vi "IMAQdxCam-Basics.vi"() -> ()   [LabVIEW 2011]
uses:
  <vilib>/vision/driver/IMAQdx.llb/IMAQdx Attribute Type.ctl
  <vilib>/vision/driver/NI_Vision_Acquisition_Software.lvlib
  C:/Program Files/National Instruments/LabVIEW 2011/resource/objmgr/imaqdx.rc
panel:
  out "Image":T1(plugin-control)
  in  "16-bit Display Mapping:Conversion Method":u32(ring)=10 items=["Default"=10, "Most Significant Bits"=11, "Full Dynamic"=12, "Downshift"=13, "Given Range"=14, "90% Dynamic"=15, "Given Percent Range"=16]
  out "LoopNo":i32
  out "error out":errorcluster
  in  "End":bool
  in  "Tab Control":enum32{"Run", "single", "startup"}(tab)=enum."startup"
  in  "Exposure":dbl(slide)=2689.598785575046 scale=100.0..100000.0
  in  "Run":bool
  in  "IMAQdx-Session":string="cam0"
  in  "AnalogGain":dbl(slide) scale=0.0..26.0
  in  "Trigger\nWait":bool
  in  "Value":dbl format="%#_9g"
  in  "Ring":u16(ring) items=["AcquisitionAttributes::AdvancedGenicam::CommandTimeout", "AcquisitionAttributes::AdvancedGenicam::EventQueueDepth", "AcquisitionAttributes::AdvancedGenicam::EventsEnabled", "AcquisitionAttributes::AdvancedGenicam::EventsSupported", "AcquisitionAttributes::Bayer::Algorithm", "AcquisitionAttributes::Bayer::GainB", "AcquisitionAttributes::Bayer::GainG", "AcquisitionAttributes::Bayer::GainR", "AcquisitionAttributes::Bayer::Pattern", "AcquisitionAttributes::ChunkDataDecoding::ChunkDataDecodingEnabled", "AcquisitionAttributes::ChunkDataDecoding::MaximumChunkCopySize", "CameraAttributes::SequencerControl::SequencerMode", "CameraAttributes::SequencerControl::SequencerSetActive", "CameraAttributes::SequencerControl::SequencerConfigurationMode", "CameraAttributes::SequencerControl::SequencerSetStart", "CameraAttributes::SequencerControl::SequencerSetSelector", "CameraAttributes::SequencerControl::SequencerSetLoad", "CameraAttributes::SequencerControl::SequencerSetSave", "CameraAttributes::SequencerControl::SequencerPathSelector", "CameraAttributes::SequencerControl::SequencerSetNext", "CameraAttributes::SequencerControl::SequencerTriggerSource", "CameraAttributes::SequencerControl::SequencerTriggerActivation", "CameraAttributes::ImageFormatControl::SensorWidth", "CameraAttributes::ImageFormatControl::SensorHeight", "CameraAttributes::ImageFormatControl::WidthMax", "CameraAttributes::ImageFormatControl::HeightMax", "CameraAttributes::ImageFormatControl::Width", "CameraAttributes::ImageFormatControl::Height", "CameraAttributes::ImageFormatControl::OffsetX", "CameraAttributes::ImageFormatControl::OffsetY", "CameraAttributes::ImageFormatControl::CenterX", "CameraAttributes::ImageFormatControl::CenterY", "CameraAttributes::ImageFormatControl::BinningHorizontalMode", "CameraAttributes::ImageFormatControl::BinningHorizontal", "CameraAttributes::ImageFormatControl::BinningVerticalMode", "CameraAttributes::ImageFormatControl::BinningVertical", "CameraAttributes::ImageFormatControl::ReverseX", "CameraAttributes::ImageFormatControl::ReverseY", "CameraAttributes::ImageFormatControl::PixelFormat", "CameraAttributes::ImageFormatControl::PixelSize", "CameraAttributes::ImageFormatControl::PixelColorFilter", "CameraAttributes::ImageFormatControl::PixelDynamicRangeMin", "CameraAttributes::ImageFormatControl::PixelDynamicRangeMax", "CameraAttributes::ImageFormatControl::TestImageSelector", "CameraAttributes::ImageFormatControl::TestImageResetAndHold", "CameraAttributes::AnalogControl::GainAuto", "CameraAttributes::AnalogControl::GainSelector", "CameraAttributes::AnalogControl::Gain", "CameraAttributes::AnalogControl::BlackLevelSelector", "CameraAttributes::AnalogControl::BlackLevel", "CameraAttributes::AnalogControl::Gamma", "CameraAttributes::AnalogControl::DigitalShift", "CameraAttributes::ImageQualityControl::PGIControl::PgiMode", "CameraAttributes::ImageQualityControl::PGIControl::NoiseReduction", "CameraAttributes::ImageQualityControl::PGIControl::SharpnessEnhancement", "CameraAttributes::ImageQualityControl::VignettingCorrectionControl::VignettingCorrectionMode", "CameraAttributes::ImageQualityControl::VignettingCorrectionControl::VignettingCorrectionLoad", "CameraAttributes::ImageQualityControl::ColorTransformationValue", "CameraAttributes::AcquisitionControl::AcquisitionMode", "CameraAttributes::AcquisitionControl::ShutterMode", "CameraAttributes::AcquisitionControl::ExposureAuto", "CameraAttributes::AcquisitionControl::ExposureMode", "CameraAttributes::AcquisitionControl::ExposureTime", "CameraAttributes::AcquisitionControl::AcquisitionBurstFrameCount", "CameraAttributes::AcquisitionControl::TriggerSelector", "CameraAttributes::AcquisitionControl::TriggerMode", "CameraAttributes::AcquisitionControl::TriggerSoftware", "CameraAttributes::AcquisitionControl::TriggerSource", "CameraAttributes::AcquisitionControl::TriggerActivation", "CameraAttributes::AcquisitionControl::TriggerDelay", "CameraAttributes::AcquisitionControl::AcquisitionFrameRateEnable", "CameraAttributes::AcquisitionControl::AcquisitionFrameRate", "CameraAttributes::AcquisitionControl::ResultingFrameRate", "CameraAttributes::AcquisitionControl::SensorReadoutTime", "CameraAttributes::AcquisitionControl::AcquisitionStatusSelector", "CameraAttributes::AcquisitionControl::AcquisitionStatus", "CameraAttributes::AutoFunctionControl::AutoTargetBrightness", "CameraAttributes::AutoFunctionControl::AutoFunctionProfile", "CameraAttributes::AutoFunctionControl::AutoGainLowerLimit", "CameraAttributes::AutoFunctionControl::AutoGainUpperLimit", "CameraAttributes::AutoFunctionControl::AutoExposureTimeLowerLimit", "CameraAttributes::AutoFunctionControl::AutoExposureTimeUpperLimit", "CameraAttributes::AutoFunctionControl::AutoFunctionROIControl::AutoFunctionROISelector", "CameraAttributes::AutoFunctionControl::AutoFunctionROIControl::AutoFunctionROIWidth", "CameraAttributes::AutoFunctionControl::AutoFunctionROIControl::AutoFunctionROIHeight", "CameraAttributes::AutoFunctionControl::AutoFunctionROIControl::AutoFunctionROIOffsetX", "CameraAttributes::AutoFunctionControl::AutoFunctionROIControl::AutoFunctionROIOffsetY", "CameraAttributes::AutoFunctionControl::AutoFunctionROIControl::AutoFunctionROIUseBrightness", "CameraAttributes::AutoFunctionControl::AutoFunctionROIControl::AutoFunctionROIUseWhiteBalance", "CameraAttributes::LUTControl::LUTSelector", "CameraAttributes::LUTControl::LUTEnable", "CameraAttributes::LUTControl::LUTIndex", "CameraAttributes::LUTControl::LUTValue", "CameraAttributes::DigitalIOControl::LineSelector", "CameraAttributes::DigitalIOControl::LineMode", "CameraAttributes::DigitalIOControl::LineFormat", "CameraAttributes::DigitalIOControl::LineLogic", "CameraAttributes::DigitalIOControl::LineSource", "CameraAttributes::DigitalIOControl::LineInverter", "CameraAttributes::DigitalIOControl::LineDebouncerTime", "CameraAttributes::DigitalIOControl::LineMinimumOutputPulseWidth", "CameraAttributes::DigitalIOControl::LineOverloadStatus", "CameraAttributes::DigitalIOControl::LineStatus", "CameraAttributes::DigitalIOControl::LineStatusAll", "CameraAttributes::DigitalIOControl::UserOutputSelector", "CameraAttributes::DigitalIOControl::UserOutputValue", "CameraAttributes::DigitalIOControl::UserOutputValueAll", "CameraAttributes::SoftwareSignalControl::SoftwareSignalSelector", "CameraAttributes::SoftwareSignalControl::SoftwareSignalPulse", "CameraAttributes::CounterAndTimerControl::TimerSelector", "CameraAttributes::CounterAndTimerControl::TimerDuration", "CameraAttributes::CounterAndTimerControl::TimerDelay", "CameraAttributes::CounterAndTimerControl::TimerTriggerSource", "CameraAttributes::CounterAndTimerControl::CounterSelector", "CameraAttributes::CounterAndTimerControl::CounterEventSource", "CameraAttributes::CounterAndTimerControl::CounterResetSource", "CameraAttributes::CounterAndTimerControl::CounterResetActivation", "CameraAttributes::CounterAndTimerControl::CounterReset", "CameraAttributes::CounterAndTimerControl::CounterDuration", "CameraAttributes::BslLightControl::BslLightControlMode", "CameraAttributes::BslLightControl::BslLightControlSource", "CameraAttributes::BslLightControl::BslLightControlEnumerateDevices", "CameraAttributes::BslLightControl::BslLightControlStatus", "CameraAttributes::BslLightControl::BslLightControlErrorStatus", "CameraAttributes::BslLightControl::BslLightControlTriggerMode", "CameraAttributes::BslLightControl::BslLightDeviceSelector", "CameraAttributes::BslLightControl::BslLightDeviceMaxCurrent", "CameraAttributes::BslLightControl::BslLightDeviceBrightness", "CameraAttributes::BslLightControl::BslLightDeviceOperationMode", "CameraAttributes::BslLightControl::BslLightDeviceStrobeMode", "CameraAttributes::BslLightControl::BslLightDeviceStrobeDuration", "CameraAttributes::BslLightControl::BslLightDeviceLastError", "CameraAttributes::BslLightControl::BslLightDeviceClearLastError", "CameraAttributes::BslLightControl::BslLightDeviceChangeID", "CameraAttributes::BslLightControl::BslLightDeviceFirmwareVersion", "CameraAttributes::ChunkDataControl::ChunkModeActive", "CameraAttributes::ChunkDataControl::ChunkSelector", "CameraAttributes::ChunkDataControl::ChunkEnable", "CameraAttributes::ChunkDataControl::ChunkGainSelector", "CameraAttributes::ChunkDataControl::ChunkGain", "CameraAttributes::ChunkDataControl::ChunkExposureTime", "CameraAttributes::ChunkDataControl::ChunkTimestamp", "CameraAttributes::ChunkDataControl::ChunkLineStatusAll", "CameraAttributes::ChunkDataControl::ChunkCounterSelector", "CameraAttributes::ChunkDataControl::ChunkCounterValue", "CameraAttributes::ChunkDataControl::ChunkSequencerSetActive", "CameraAttributes::ChunkDataControl::ChunkPayloadCRC16", "CameraAttributes::ChunkDataControl::ChunkData::ChunkGainSelector", "CameraAttributes::ChunkDataControl::ChunkData::ChunkGain", "CameraAttributes::ChunkDataControl::ChunkData::ChunkExposureTime", "CameraAttributes::ChunkDataControl::ChunkData::ChunkTimestamp", "CameraAttributes::ChunkDataControl::ChunkData::ChunkLineStatusAll", "CameraAttributes::ChunkDataControl::ChunkData::ChunkCounterSelector", "CameraAttributes::ChunkDataControl::ChunkData::ChunkCounterValue", "CameraAttributes::ChunkDataControl::ChunkData::ChunkSequencerSetActive", "CameraAttributes::ChunkDataControl::ChunkData::ChunkPayloadCRC16", "CameraAttributes::EventControl::EventSelector", "CameraAttributes::EventControl::EventNotification", "CameraAttributes::EventControl::EventExposureEndData::EventExposureEnd", "CameraAttributes::EventControl::EventExposureEndData::EventExposureEndTimestamp", "CameraAttributes::EventControl::EventExposureEndData::EventExposureEndFrameID", "CameraAttributes::EventControl::EventFrameBurstStartData::EventFrameBurstStart", "CameraAttributes::EventControl::EventFrameBurstStartData::EventFrameBurstStartTimestamp", "CameraAttributes::EventControl::EventFrameBurstStartData::EventFrameBurstStartFrameID", "CameraAttributes::EventControl::EventFrameStartOvertriggerData::EventFrameStartOvertrigger", "CameraAttributes::EventControl::EventFrameStartOvertriggerData::EventFrameStartOvertriggerTimestamp", "CameraAttributes::EventControl::EventFrameStartOvertriggerData::EventFrameStartOvertriggerFrameID", "CameraAttributes::EventControl::EventFrameBurstStartOvertriggerData::EventFrameBurstStartOvertrigger", "CameraAttributes::EventControl::EventFrameBurstStartOvertriggerData::EventFrameBurstStartOvertriggerTimestamp", "CameraAttributes::EventControl::EventFrameBurstStartOvertriggerData::EventFrameBurstStartOvertriggerFrameID", "CameraAttributes::EventControl::EventCriticalTemperatureData::EventCriticalTemperature", "CameraAttributes::EventControl::EventCriticalTemperatureData::EventCriticalTemperatureTimestamp", "CameraAttributes::EventControl::EventOverTemperatureData::EventOverTemperature", "CameraAttributes::EventControl::EventOverTemperatureData::EventOverTemperatureTimestamp", "CameraAttributes::EventControl::EventFrameStartWaitData::EventFrameStartWait", "CameraAttributes::EventControl::EventFrameStartWaitData::EventFrameStartWaitTimestamp", "CameraAttributes::EventControl::EventFrameBurstStartWaitData::EventFrameBurstStartWait", "CameraAttributes::EventControl::EventFrameBurstStartWaitData::EventFrameBurstStartWaitTimestamp", "CameraAttributes::UserSetControl::UserSetSelector", "CameraAttributes::UserSetControl::UserSetLoad", "CameraAttributes::UserSetControl::UserSetSave", "CameraAttributes::UserSetControl::UserSetDefault", "CameraAttributes::TransportLayerControl::PayloadSize", "CameraAttributes::TransportLayerControl::BslUSBSpeedMode", "CameraAttributes::TransportLayerControl::SIPayloadTransferSize", "CameraAttributes::TransportLayerControl::SIPayloadTransferCount", "CameraAttributes::TransportLayerControl::SIPayloadFinalTransfer1Size", "CameraAttributes::TransportLayerControl::SIPayloadFinalTransfer2Size", "CameraAttributes::DeviceControl::DeviceVendorName", "CameraAttributes::DeviceControl::DeviceModelName", "CameraAttributes::DeviceControl::DeviceManufacturerInfo", "CameraAttributes::DeviceControl::DeviceVersion", "CameraAttributes::DeviceControl::DeviceFirmwareVersion", "CameraAttributes::DeviceControl::DeviceSerialNumber", "CameraAttributes::DeviceControl::DeviceUserID", "CameraAttributes::DeviceControl::DeviceScanType", "CameraAttributes::DeviceControl::TimestampLatch", "CameraAttributes::DeviceControl::TimestampLatchValue", "CameraAttributes::DeviceControl::DeviceLinkSelector", "CameraAttributes::DeviceControl::DeviceLinkSpeed", "CameraAttributes::DeviceControl::DeviceLinkThroughputLimitMode", "CameraAttributes::DeviceControl::DeviceLinkThroughputLimit", "CameraAttributes::DeviceControl::DeviceLinkCurrentThroughput", "CameraAttributes::DeviceControl::DeviceTemperatureSelector", "CameraAttributes::DeviceControl::DeviceTemperature", "CameraAttributes::DeviceControl::TemperatureState", "CameraAttributes::DeviceControl::DeviceSFNCVersionMajor", "CameraAttributes::DeviceControl::DeviceSFNCVersionMinor", "CameraAttributes::DeviceControl::DeviceSFNCVersionSubMinor", "CameraAttributes::UserDefinedValueControl::UserDefinedValueSelector", "CameraAttributes::UserDefinedValueControl::UserDefinedValue", "CameraAttributes::RemoveParameterLimitControl::RemoveParameterLimitSelector", "CameraAttributes::RemoveParameterLimitControl::RemoveParameterLimit", "CameraAttributes::ExpertFeatureAccess::ExpertFeatureAccessSelector", "CameraAttributes::ExpertFeatureAccess::ExpertFeatureAccessKey", "CameraAttributes::ExpertFeatureAccess::ExpertFeatureEnable", "CameraAttributes::FileAccessControl::FileSelector", "CameraAttributes::FileAccessControl::FileOperationSelector", "CameraAttributes::FileAccessControl::FileOpenMode", "CameraAttributes::FileAccessControl::FileAccessOffset", "CameraAttributes::FileAccessControl::FileAccessLength", "CameraAttributes::FileAccessControl::FileOperationStatus", "CameraAttributes::FileAccessControl::FileOperationResult", "CameraAttributes::FileAccessControl::FileSize", "CameraAttributes::FileAccessControl::FileOperationExecute", "AcquisitionAttributes::BitsPerPixel", "AcquisitionAttributes::ImageDecoderCopyMode", "AcquisitionAttributes::IncompleteBufferMode", "AcquisitionAttributes::OutputImageType", "AcquisitionAttributes::OverwriteMode", "AcquisitionAttributes::ReceiveTimestampMode", "AcquisitionAttributes::ShiftPixelBits", "AcquisitionAttributes::SwapPixelBytes", "AcquisitionAttributes::Timeout", "CameraInformation::BaseAddress", "CameraInformation::BusType", "CameraInformation::ModelName", "CameraInformation::PrimaryURLString", "CameraInformation::SecondaryURLString", "CameraInformation::SerialNumberHigh", "CameraInformation::SerialNumberLow", "CameraInformation::USBConnectionSpeed", "CameraInformation::VendorName", "StatusInformation::AcqInProgress", "StatusInformation::HandledEventCount", "StatusInformation::IncompleteBufferCount", "StatusInformation::LastBufferCount", "StatusInformation::LastBufferNumber", "StatusInformation::LostBufferCount", "StatusInformation::LostEventCount"]
  out "Description":string
  out "IsWritable":bool
  out "Attribute Type":T2=enum."Bool"
  in  "IMAQdx-start":string
  out "initerror":errorcluster
  # "init an test the cam with NiMax first! Find Session name"
  # "! Space nach name und type vor komma\nName, \nType[U32,I64,DBL,String,Enum,Bool,Command], \nRead, \nWrite[0,1], \nValue"
  # "init the cam in MAX first!"
  # "read"
  # "change=write"
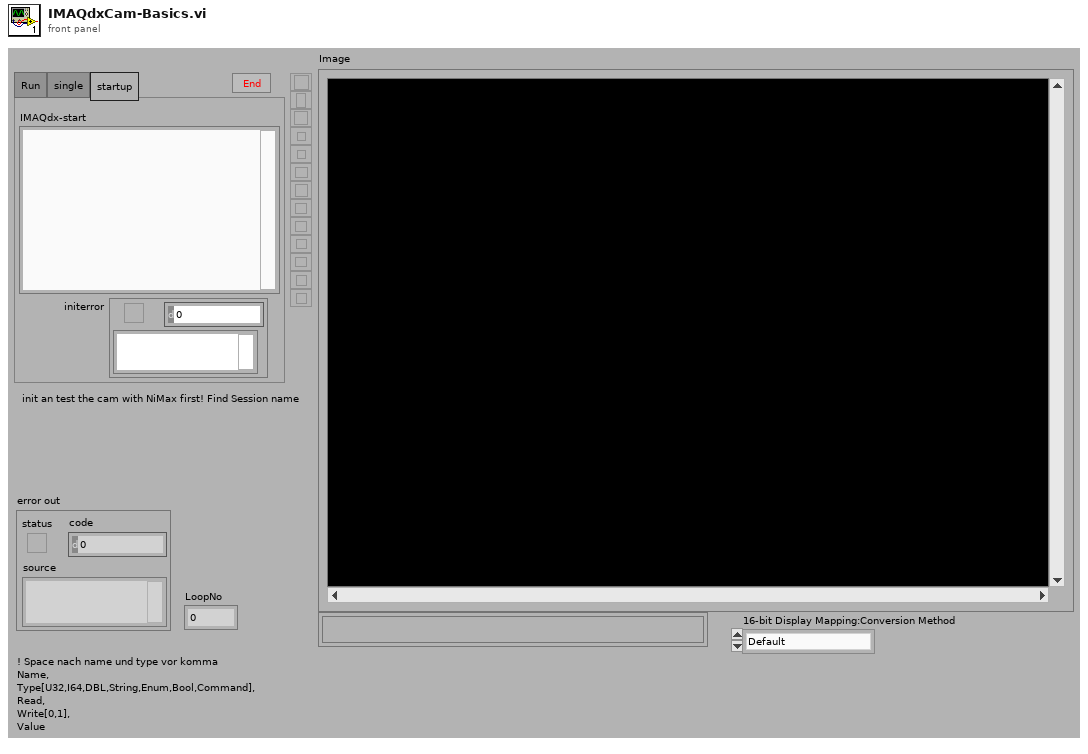
[diagram p1: front panel]
types:
  T1 = typedef "IMAQ Image.ctl" = refnum<image>
  T2 = typedef "NI_Vision_Acquisition_Software.lvlib/IMAQdx Attribute Type.ctl" = enum32{"U32", "I64", "DBL", "String", "Enum", "Bool", "Command"}
  T3 = typedef "Image Type" = u32
  T4 = typedef "IMAQdx.ctl" = refnum<k21>
  T5 = cluster{"Attribute Type":T2, "Readable":bool, "Writable":bool, "Attribute Name":string}[]
  T6 = cluster{"Global Rectangle":i32[], "Contours":cluster{"Contour Type":u32, "ROI Type":u32, "Points":i32[]}[]}
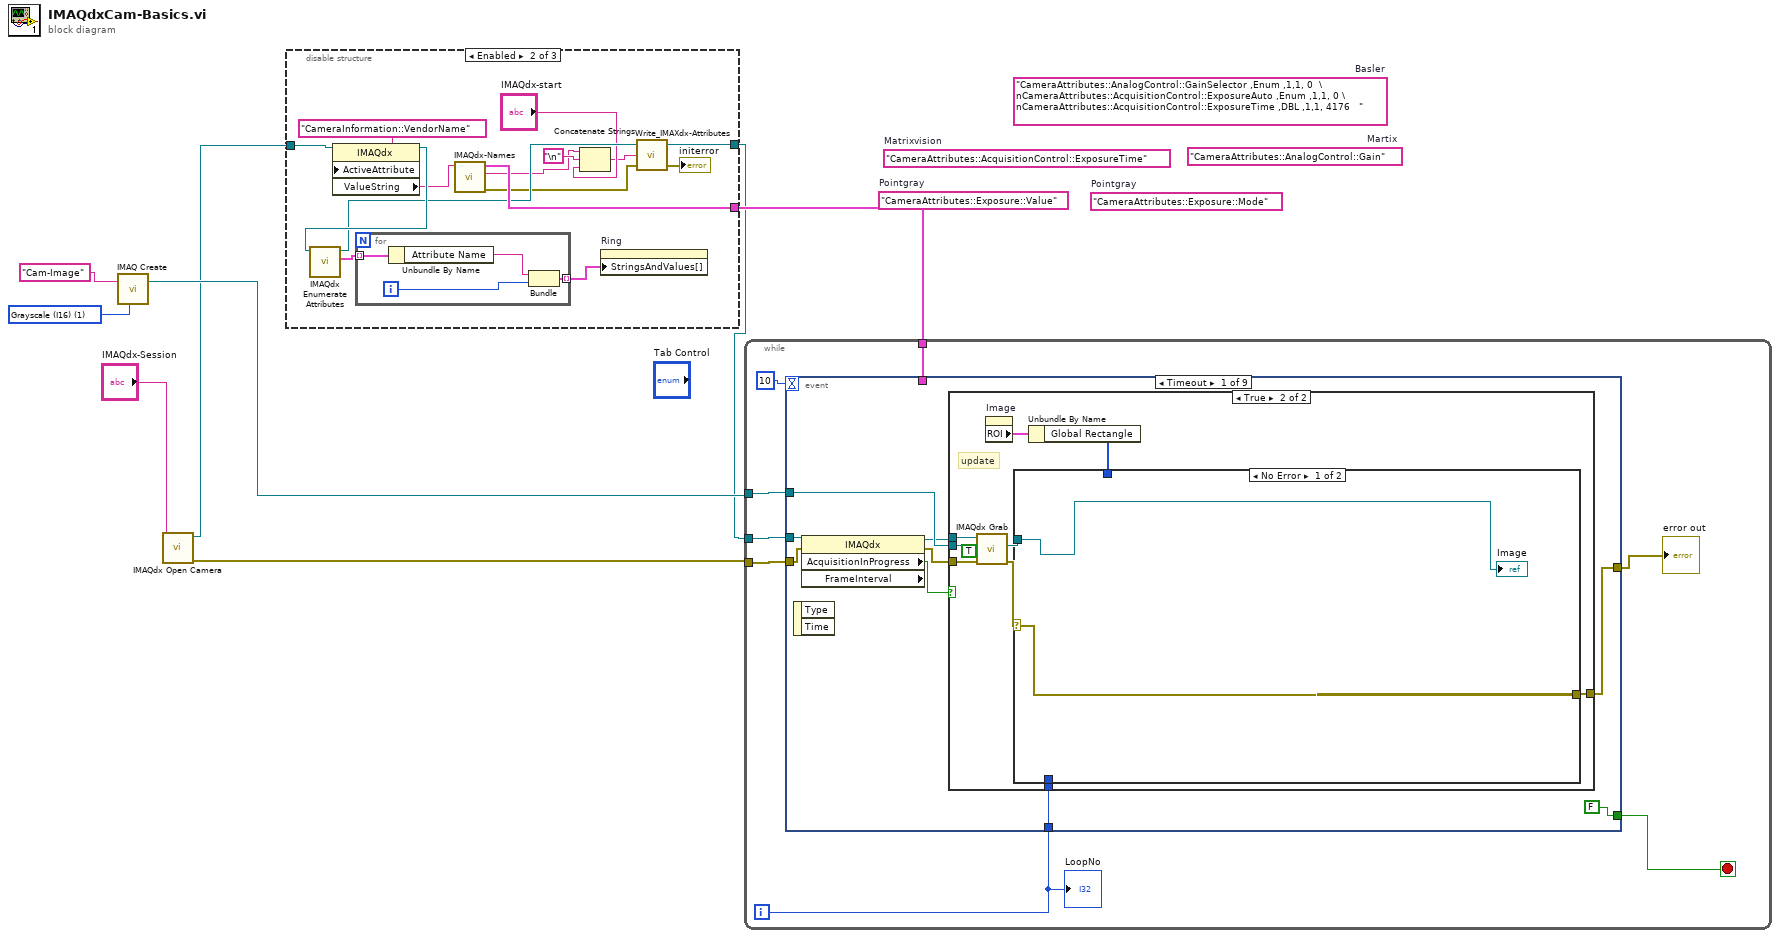
[diagram p0: block diagram]
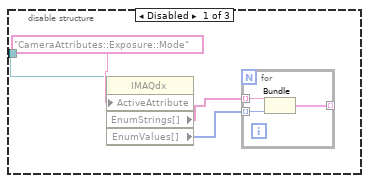
[diagram p2: hidden frame]
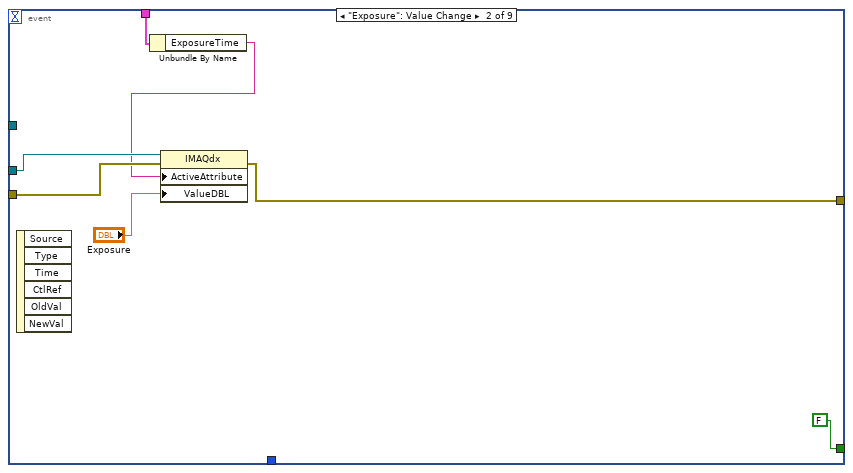
[diagram p6: hidden frame]
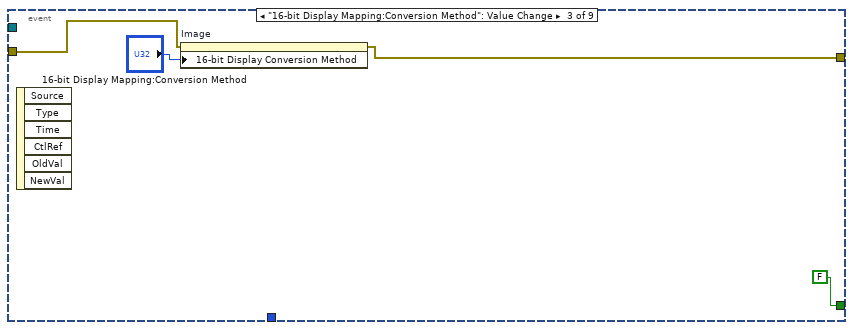
[diagram p7: hidden frame]
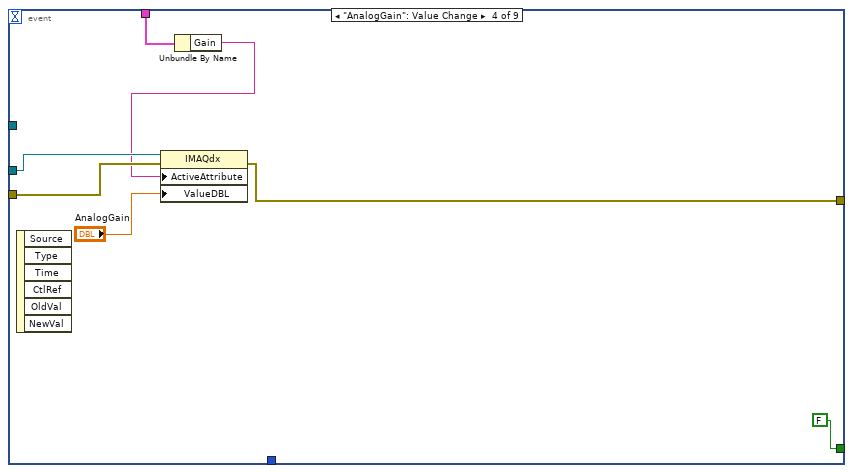
[diagram p8: hidden frame]
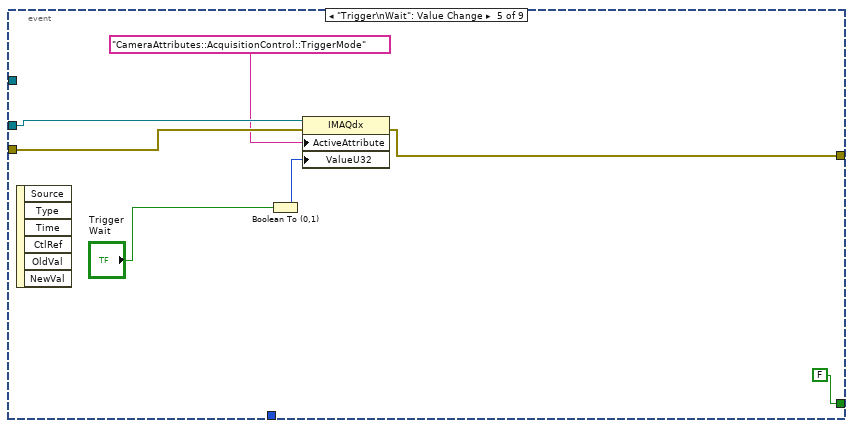
[diagram p9: hidden frame]
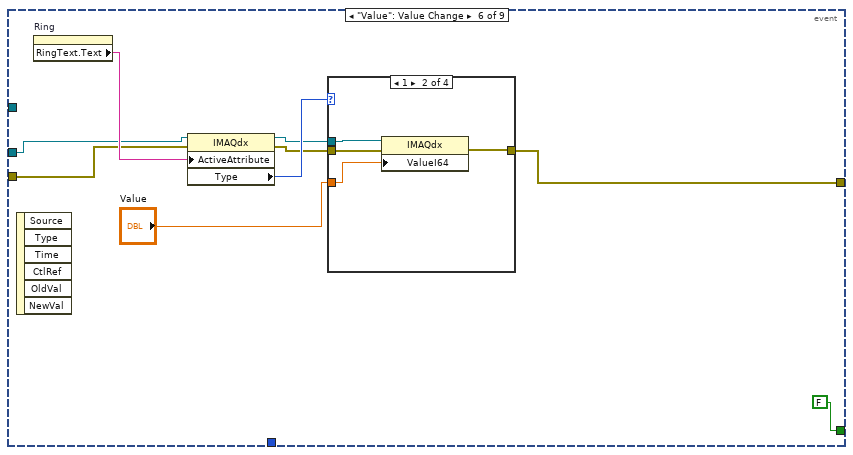
[diagram p10: hidden frame]
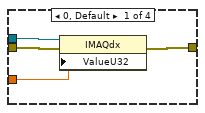
[diagram p11: hidden frame]
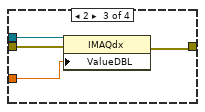
[diagram p12: hidden frame]
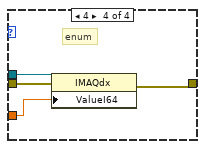
[diagram p13: hidden frame]
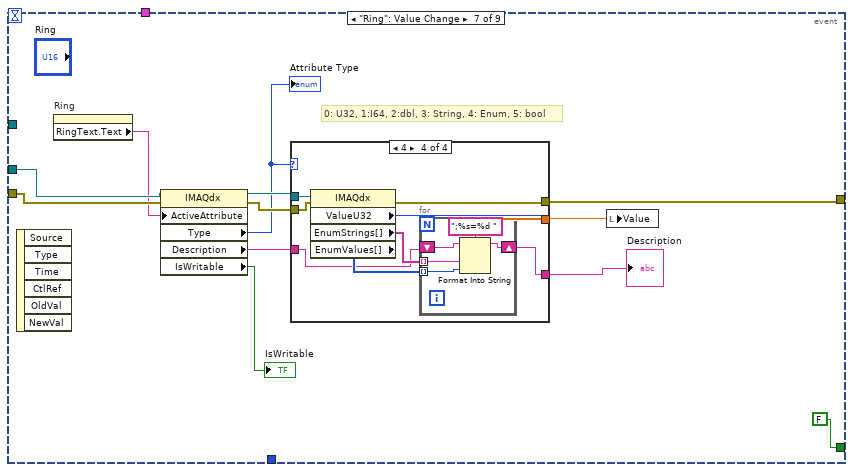
[diagram p14: hidden frame]
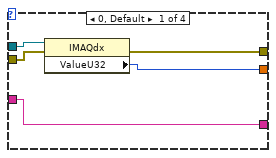
[diagram p15: hidden frame]
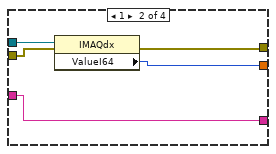
[diagram p16: hidden frame]
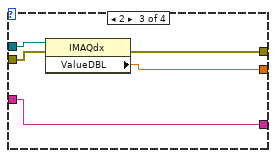
[diagram p17: hidden frame]
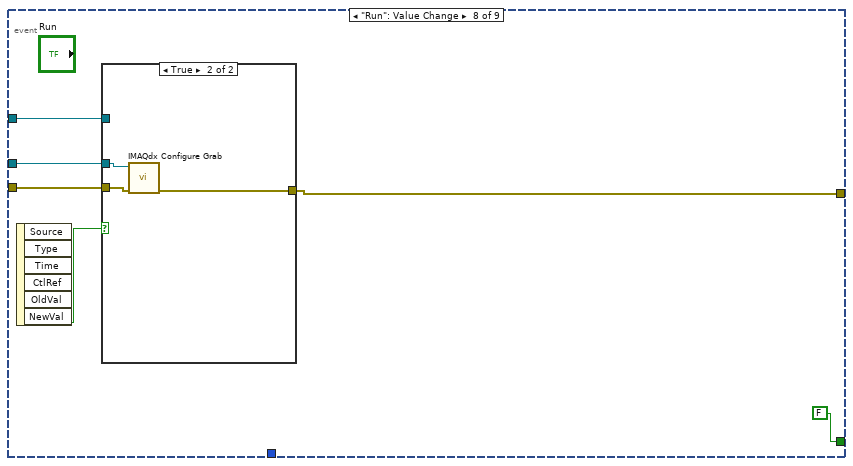
[diagram p18: hidden frame]
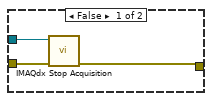
[diagram p19: hidden frame]
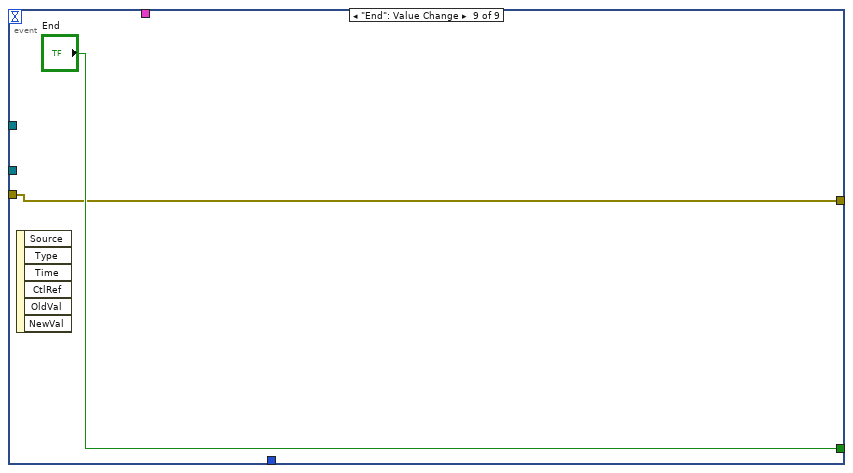
[diagram p20: hidden frame]
diagram:
  (unwired) "CameraAttributes::AnalogControl::Gain"  # Martix
  (unwired) "CameraAttributes::AnalogControl::GainSelector ,Enum ,1,1, 0  \nCameraAttributes::AcquisitionControl::ExposureAuto ,Enum ,1,1, 0 \nCameraAttributes::AcquisitionControl::ExposureTime ,DBL ,1,1, 4176   "  # Basler
  (unwired) "CameraAttributes::Exposure::Mode"  # Pointgray
  (unwired) "CameraAttributes::Exposure::Value"  # Pointgray
  (unwired) "CameraAttributes::AcquisitionControl::ExposureTime"  # Matrixvision
  w3 = T3 1 items=["Grayscale (U8)", "Grayscale (I16)", "Grayscale (SGL)", "Complex (CSG)", "RGB (U32)", "HSL (U32)", "RGB (U64)", "Grayscale (U16)"] ("Image Type")
  n1 = call "IMAQ Create"("Image Name"="Cam-Image", "Image Type"=w3) -> ("New Image"=w6:T1)  [unwired: 2 in, 2 out]
  n2 = call <vilib>:"IMAQdx Open Camera.vi"("Session In"="IMAQdx-Session") -> ("error out"=w7:errorcluster, "Session Out"=w5:T4)  [unwired: 2 in, 7 out]
  n3 = disable-structure shown="Enabled" {
    disable-tunnel: w5 -> [w11 w28 w35]
    disable-tunnel: [_ w24 _] -> w2
    disable-tunnel: [_ w22 w35] -> w1
    frame Disabled {
      n4 = property class="IMAQdx"(reference=w11, "ActiveAttribute"="CameraAttributes::Exposure::Mode" ("Attribute Name")) -> ("EnumStrings[]"=w10:string[], "EnumValues[]"=w9:u32[])  [unwired: 1 in, 2 out]
      n5 = for {
        tunnel: w10 -> [w15] mode=indexing
        tunnel: w9 -> [w14] mode=indexing
        tunnel: [w13] -> _ mode=indexing
        n6 = Bundle(w15, w14) -> (w13:cluster{string, u32})  [unwired: 1 out]
      }
    }
    frame Enabled {
      n7 = property class="IMAQdx"(reference=w28, "ActiveAttribute"="CameraInformation::VendorName") -> (reference out=w26:T4, "ValueString"=w25:string)  [unwired: 1 in, 1 out]
      n8 = call <vilib>:"IMAQdx Enumerate Attributes.vi"("Session In"=w26) -> ("Attribute Information Array"=w27:T5, "Session Out"=w23:T4)  [unwired: 8 in, 1 out]
      n9 = for {
        tunnel: w27 -> [w34] mode=indexing
        tunnel: [w31] -> w29 mode=indexing
        i -> [w32]
        n10 = Unbundle By Name(w34) -> ("Attribute Name"=w33:string)
        n11 = Bundle("Attribute Name"=w33, w32) -> (w31:cluster{"Attribute Name":string, i32})  [unwired: 1 in]
      }
      n12 = call "IMAQdx-Names.vi"("exactCameraName"=w25) -> ("error out"=w16:errorcluster, "Defaults"=w20:string, "shortcuts"=w24:cluster{"ExposureTime":string, "Gain":string})  [unwired: 8 in]
      n13 = Concatenate Strings(w20, "\n", "IMAQdx-start") -> (w18:string)
      n14 = property on="Ring" class="Ring (strict)"("StringsAndValues[]"=w29) -> ()  [unwired: 2 in, 2 out]
      n15 = call "Write_IMAXdx-Attributes.vi"("error in"=w16, "IMAQdx-Defaults"=w18, "Session In"=w23) -> ("error out"=→"initerror":errorcluster, "Session Out"=w22:T4)  [unwired: 1 in]
    }
    frame Disabled {
    }
  }
  n16 = while {
    tunnel: w1 -> [w43]
    tunnel: w7 -> [w42]
    tunnel: w6 -> [w41]
    tunnel: w2 -> [w36]
    i -> [w37]
    stop <- w40 stop-if-true
    n17 = event shown="[0] Timeout" {
      selector: _ -> [_ _ _ _ _ _ _ _ _]
      dyn-events: _ -> [_ _ _ _ _ _ _ _ _]
      timeout: 10 -> [_ _ _ _ _ _ _ _ _]
      tunnel: w43 -> [w48 w72 _ w84 w89 w96 w126 w161 _]
      tunnel: w42 -> [w47 w71 w75 w83 w88 w94 w124 w160 w169]
      tunnel: w41 -> [w52 _ _ _ _ _ _ w159 _]
      tunnel: [FALSE ("End") FALSE ("End") FALSE ("End") FALSE ("End") FALSE ("End") FALSE ("End") FALSE ("End") FALSE ("End") "End"] -> w40
      tunnel: [w49 w70 w74 w82 w86 w100 w128 w158 w169] -> w38
      tunnel: w37 -> [w45 _ _ _ _ _ _ _ _]
      tunnel: w36 -> [_ w69 _ w81 _ _ _ _ _]
      event Timeout {
        n18 = event-data() -> ()  [unwired: 3 out]
        n19 = property class="IMAQdx" props=["AcquisitionInProgress", "FrameInterval"](reference=w48, error in=w47) -> (reference out=w50:T4, error out=w46:errorcluster, "AcquisitionInProgress"=w51:bool)  [unwired: 1 out]
        n20 = case shown="True" w51 {
          tunnel: w52 -> [_ w63]
          tunnel: w46 -> [w53 w62]
          tunnel: w50 -> [_ w61]
          tunnel: [w53 w57] -> w49
          tunnel: w45 -> [_ w58]
          frame False {
          }
          frame True {
            # "update"
            n21 = call <vilib>:"IMAQdx Grab.vi"("error in"=w62, "Wait for Next Buffer? (Yes)"=TRUE, "Image In"=w63, "Session In"=w61) -> ("error out"=w55:errorcluster, "Image Out"=w59:T1)  [unwired: 6 out]
            n22 = property on="Image" class="ImageControl"() -> ("ROI"=w54:T6)  [unwired: 2 in, 2 out]
            n23 = Unbundle By Name(w54) -> ("Global Rectangle"=w56:i32[])
            n24 = case shown="No Error" w55 {
              selector: w55 -> [w65 w66]
              tunnel: w59 -> [w64 _]
              tunnel: w58 -> [_ _]
              tunnel: [w65 w66] -> w57
              tunnel: w56 -> [_ _]
              frame No Error {
                "Image" <- w64
              }
              frame Error {
              }
            }
          }
        }
      }
      event "Exposure": Value Change {
        n25 = event-data() -> ()  [unwired: 7 out]
        n26 = Unbundle By Name(w69) -> ("ExposureTime"=w68:string)
        n27 = property class="IMAQdx"(reference=w72, error in=w71, "ActiveAttribute"=w68, "ValueDBL"="Exposure") -> (error out=w70:errorcluster)  [unwired: 1 out]
      }
      event "16-bit Display Mapping:Conversion Method": Value Change {
        n28 = event-data() -> ()  [unwired: 7 out]
        n29 = property on="Image" class="ImageControl"(error in=w75, "16-bit Display Conversion Method"="16-bit Display Mapping:Conversion Method") -> (error out=w74:errorcluster)  [unwired: 1 in, 1 out]
      }
      event "AnalogGain": Value Change {
        n30 = event-data() -> ()  [unwired: 7 out]
        n31 = Unbundle By Name(w81) -> ("Gain"=w80:string)
        n32 = property class="IMAQdx"(reference=w84, error in=w83, "ActiveAttribute"=w80, "ValueDBL"="AnalogGain") -> (error out=w82:errorcluster)  [unwired: 1 out]
      }
      event "Trigger\nWait": Value Change {
        n33 = event-data() -> ()  [unwired: 7 out]
        n34 = Boolean To (0,1)(Boolean="Trigger\nWait") -> (0, 1=w91:i16)
        n35 = property class="IMAQdx"(reference=w89, error in=w88, "ActiveAttribute"="CameraAttributes::AcquisitionControl::TriggerMode", "ValueU32"=w91) -> (error out=w86:errorcluster)  [unwired: 1 out]
      }
      event "Value": Value Change {
        n36 = event-data() -> ()  [unwired: 7 out]
        n37 = property on="Ring" class="Ring (strict)"() -> ("RingText.Text"=w98:string)  [unwired: 2 in, 2 out]
        n38 = property class="IMAQdx"(reference=w96, error in=w94, "ActiveAttribute"=w98) -> (reference out=w95:T4, error out=w93:errorcluster, "Type"=w97:u32)
        n39 = case shown="1" w97 {
          tunnel: w95 -> [w104 w108 w112 w116]
          tunnel: w93 -> [w103 w105 w111 w115]
          tunnel: [w102 w106 w110 w114] -> w100
          tunnel: "Value" -> [w101 w107 w109 w113]
          frame 0, Default {
            n40 = property class="IMAQdx"(reference=w104, error in=w103, "ValueU32"=w101) -> (error out=w102:errorcluster)  [unwired: 1 out]
          }
          frame 1 {
            n41 = property class="IMAQdx"(reference=w108, error in=w105, "ValueI64"=w107) -> (error out=w106:errorcluster)  [unwired: 1 out]
          }
          frame 2 {
            n42 = property class="IMAQdx"(reference=w112, error in=w111, "ValueDBL"=w109) -> (error out=w110:errorcluster)  [unwired: 1 out]
          }
          frame 4 {
            # "enum"
            n43 = property class="IMAQdx"(reference=w116, error in=w115, "ValueI64"=w113) -> (error out=w114:errorcluster)  [unwired: 1 out]
          }
        }
      }
      event "Ring": Value Change {
        # "0: U32, 1:I64, 2:dbl, 3: String, 4: Enum, 5: bool"
        n44 = event-data() -> ()  [unwired: 7 out]
        n45 = property on="Ring" class="Ring (strict)"() -> ("RingText.Text"=w122:string)  [unwired: 2 in, 2 out]
        n46 = property class="IMAQdx"(reference=w126, error in=w124, "ActiveAttribute"=w122) -> (reference out=w125:T4, error out=w123:errorcluster, "Type"=w119:u32, "Description"=w118:string, "IsWritable"=→"IsWritable":bool)
        "Attribute Type" <- w119
        n47 = case shown="4" w119 {
          tunnel: w123 -> [w132 w137 w142 w150]
          tunnel: w125 -> [w133 w138 w143 w151]
          tunnel: [w131 w136 w140 w149] -> w128
          tunnel: [w130 w135 w141 w148] -> w127
          tunnel: [w129 w134 w139 w145] -> w117
          tunnel: w118 -> [w129 w134 w139 w144]
          frame 0, Default {
            n48 = property class="IMAQdx"(reference=w133, error in=w132) -> (error out=w131:errorcluster, "ValueU32"=w130:u32)  [unwired: 1 out]
          }
          frame 1 {
            n49 = property class="IMAQdx"(reference=w138, error in=w137) -> (error out=w136:errorcluster, "ValueI64"=w135:i64)  [unwired: 1 out]
          }
          frame 2 {
            n50 = property class="IMAQdx"(reference=w143, error in=w142) -> (error out=w140:errorcluster, "ValueDBL"=w141:dbl)  [unwired: 1 out]
          }
          frame 4 {
            n51 = property class="IMAQdx"(reference=w151, error in=w150) -> (error out=w149:errorcluster, "ValueU32"=w148:u32, "EnumStrings[]"=w147:string[], "EnumValues[]"=w146:u32[])  [unwired: 1 out]
            n52 = for {
              tunnel: w147 -> [w156] mode=indexing
              tunnel: w146 -> [w155] mode=indexing
              shift-right: [w153] -> w145
              shift-left: w144 -> [w154]
              n53 = Format Into String(format string=";%s=%d ", initial string=w154, w156, w155) -> (resulting string=w153:string)  [unwired: 1 in, 1 out]
            }
          }
        }
        "Description" <- w117
        n54 = local write "Value"(w127) -> ()
      }
      event "Run": Value Change {
        n55 = event-data() -> ("NewVal"=w162:bool)  [unwired: 6 out]
        n56 = case shown="True" w162 {
          tunnel: w161 -> [w165 w168]
          tunnel: w160 -> [w164 w167]
          tunnel: w159 -> [_ _]
          tunnel: [w163 w166] -> w158
          frame False {
            n57 = call <vilib>:"IMAQdx Stop Acquisition.vi"("error in"=w164, "Session In"=w165) -> ("error out"=w163:errorcluster)  [unwired: 9 out]
          }
          frame True {
            n58 = call <vilib>:"IMAQdx Configure Grab.vi"("error in"=w167, "Session In"=w168) -> ("error out"=w166:errorcluster)  [unwired: 9 out]
          }
        }
      }
      event "End": Value Change {
        n59 = event-data() -> ()  [unwired: 7 out]
      }
    }
    "error out" <- w38
    "LoopNo" <- w37
  }
